vi "FILE PATH CREATION Unitest.vi"(8 "error in":errorcluster, 11 "FILE NAME :":string) -> (0 "error out":errorcluster, 3 "FILE OUT":path)   [LabVIEW 2025]
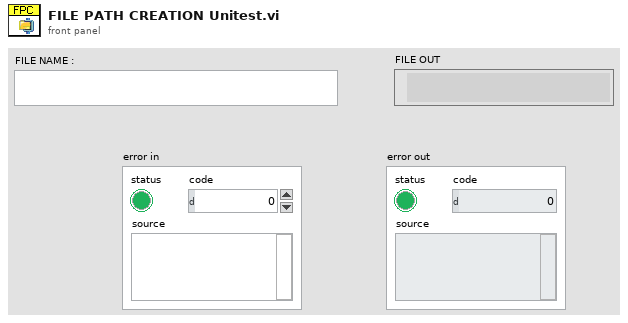
[diagram p1: front panel]
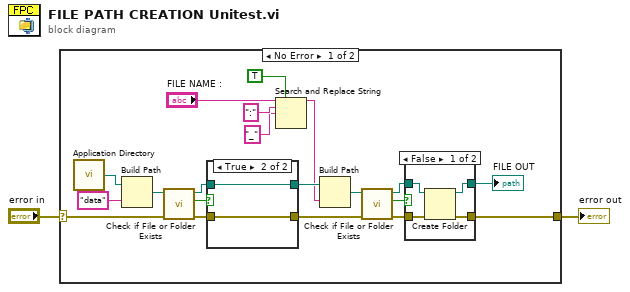
[diagram p0: block diagram]
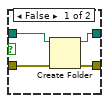
[diagram p3: hidden frame]
diagram:
  n1 = case shown="No Error" "error in" {
    selector: "error in" -> [w11 _]
    tunnel: [w13 _] -> w2
    frame No Error {
      n2 = call <vilib>:"Application Directory.vi"() -> ("Application Directory"=w10:path)
      n3 = Build Path(base path=w10, name or relative path="data") -> (appended path=w3:path)
      n4 = call <vilib>:"Check if File or Folder Exists.vi"("error in (no error)"=w11, "path"=w3) -> ("error out"=w19:errorcluster, "file or folder exists?"=w21:bool, "dup path"=w20:path)  [unwired: 7 in]
      n5 = case shown="True" w21 {
        tunnel: w20 -> [w32 w33]
        tunnel: w19 -> [w31 w34]
        tunnel: [w30 w34] -> w12
        tunnel: [w29 w33] -> w18
        frame False {
          n6 = Create Folder(path (use dialog)=w32, error in=w31) -> (created path=w29:path, error out=w30:errorcluster)  [unwired: 1 in, 1 out]
        }
        frame True {
        }
      }
      n7 = Search and Replace String(replace all?=TRUE ("replace all? (F)"), input string="FILE NAME :", search string=":", replace string="_" ("replace string (\"\")")) -> (result string=w5:string)  [unwired: 4 in, 3 out]
      n8 = Build Path(base path=w18, name or relative path=w5) -> (appended path=w14:path)
      n9 = call <vilib>:"Check if File or Folder Exists.vi"("error in (no error)"=w12, "path"=w14) -> ("error out"=w17:errorcluster, "file or folder exists?"=w15:bool, "dup path"=w16:path)  [unwired: 7 in]
      n10 = case shown="False" w15 {
        tunnel: w16 -> [w26 w27]
        tunnel: w17 -> [w25 w28]
        tunnel: [w24 w28] -> w13
        tunnel: [w23 w27] -> w9
        frame False {
          n11 = Create Folder(path (use dialog)=w26, error in=w25) -> (created path=w23:path, error out=w24:errorcluster)  [unwired: 1 in, 1 out]
        }
        frame True {
        }
      }
      "FILE OUT" <- w9
    }
    frame Error {
    }
  }
  "error out" <- w2
